vi "Connect-Disconnect.vi"(8 "Error In":errorcluster) -> (0 "Error Out":errorcluster)   [LabVIEW 2017, in "Tests.lvlib" / "Session.lvlib"]
uses:
  Session.lvlib
  src/LabSSH2/LabSSH2.lvlib
  src/LabSSH2/Public/SSH/Session.lvclass
  <vilib>/addons/_JKI Toolkits/Caraya/classes/Test/Test.lvclass
  <vilib>/addons/_JKI Toolkits/Caraya/classes/Assert/Assert.lvclass
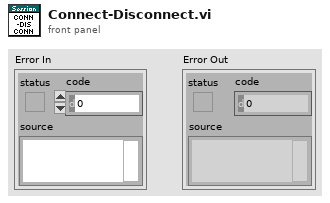
[diagram p1: front panel]
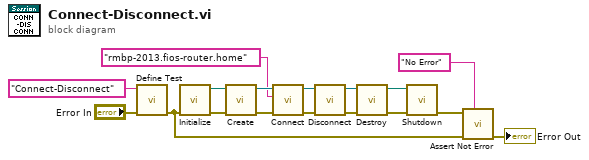
[diagram p0: block diagram]
diagram:
  n1 = call <vilib>:"Define Test.vi"("error in (no error)"="Error In", "Label (VI Title)"="Connect-Disconnect") -> ("error out"=w12:errorcluster)  [unwired: 9 in]
  n2 = call "Initialize.vi"("Error In"=w12) -> ("Error Out"=w16:errorcluster, "labssh2 Shared Library Out"=w8:path)  [unwired: 9 in]
  n3 = call "Create.vi"("Error In"=w16, "labssh2 Shared Library"=w8) -> ("Error Out"=w6:errorcluster, "Sesssion"=w7:refnum<class "Session.lvclass">)  [unwired: 8 in]
  n4 = call "Connect.vi"("Error In"=w6, "Address"="rmbp-2013.fios-router.home", "Session In"=w7) -> ("Error Out"=w2:errorcluster, "Sesssion Out"=w5:refnum<class "Session.lvclass">)  [unwired: 7 in]
  n5 = call "Disconnect.vi"("Error In"=w2, "Session In"=w5) -> ("Error Out"=w3:errorcluster, "Sesssion Out"=w4:refnum<class "Session.lvclass">)  [unwired: 8 in]
  n6 = call "Destroy.vi"("Error In"=w3, "Session"=w4) -> ("Error Out"=w14:errorcluster, "labssh2 Shared Library"=w15:path)  [unwired: 8 in]
  n7 = call "Shutdown.vi"("Error In"=w14, "labssh2 Shared Library"=w15) -> ("Error Out"=w13:errorcluster)  [unwired: 9 in]
  n8 = call <vilib>:"Assert Not Error.vi"("Label"="No Error", "error in (no error)"=w12, "Not Error?"=w13) -> ("error out"=→"Error Out":errorcluster)  [unwired: 8 in]
